vi "Actor Core.vi"(8 "error in":errorcluster, 11 "Nested in":refnum<class "FlatFieldUI.lvclass">) -> (0 "error out":errorcluster, 3 "Actor out":refnum<class "Actor.lvclass">)   [LabVIEW 2020, in "FlatField.lvlib" / "FlatFieldUI.lvlib" / "FlatFieldUI.lvclass"]
doc: "(<B>Filename</B>: Actor Framework.lvlib:Actor.lvclass:Actor Core.vi)\n\nReceives messages to the actor, reacts to them, and initiates any error handling that may shut the actor down.\n\nDescendant classes may override this VI to append parallel tasks for the actor to complete while it handles messages. Overrides use the Call Parent Method node."
uses:
  FlatFieldUI.lvclass
  C:/Program Files/National Instruments/LabVIEW 2020/vi.lib/ActorFramework/Actor/Actor.lvclass
  <vilib>/ActorFramework/Actor/Actor.lvclass
  Displayer/Displayer/FlatField Method.ctl
  FlatFieldUI.lvclass/FlatFieldUI.ctl
  <vilib>/ActorFramework/Actor/Actor.lvclass/Actor.ctl
  <vilib>/ActorFramework/Message Enqueuer/Message Enqueuer.lvclass/Message Enqueuer.ctl
  Model/Hardware Abstraction Layer/Component/Device/Device/DataExchange.ctl
  Interface/DataListener Messages/OnDataChange Msg/OnDataChange Msg.lvclass/OnDataChange Msg.ctl
  <vilib>/ActorFramework/Message Enqueuer/Init from Existing Queue.vi
  <vilib>/ActorFramework/Message Enqueuer/Enqueue.vi
  Interface/DataListener Messages/OnDataChange Msg/OnDataChange Msg.lvclass
  C:/Program Files/National Instruments/LabVIEW 2020/vi.lib/ActorFramework/Message/Message.lvclass
  <vilib>/ActorFramework/Stop Msg/Stop Msg.lvclass
  <vilib>/ActorFramework/Message Priority Queue/Priority Enqueue.vi
  <vilib>/ActorFramework/Message Enqueuer/Message Enqueuer.lvclass
  Interface/DataListener/DataListener.lvclass
  FlatField/FlatField/FlatField.lvclass
panel:
  in  "FlatFieldPath":path
  in  "DarkFieldPath":path
  in  "Save FlatField Image":bool
  in  "Save DarkField Image":bool
  in  "Method":T1 items=["Average", "Median"]
  out "Waveform Chart":dbl(graph)
  in  "Show FlatField Image":bool
  in  "Show DarkField Image":bool
  out "Frames/Dark Field":dbl
  out "Frames/Flat-Field":dbl
  in  "Frames/Flat-Field":dbl
  in  "Frames/Dark Field":dbl
  in  "TakeFlatFieldImage":bool
  in  "TakeDarkFieldImage":bool
  out "RawImage":T2(plugin-control)
  in  "Flat-Field":bool
  # "* Please Take DarkField & Flat Field Images In Live Mode\n* You need to save the DarkField/FlatField images manually for post-processing"
  # "/"
  # "1."
  # "/"
  # "2."
  # "3."
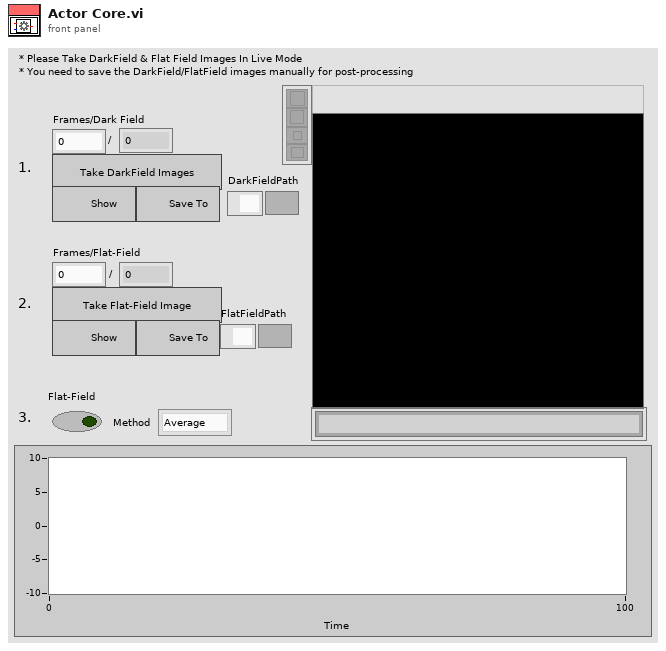
[diagram p1: front panel]
types:
  T1 = typedef "FlatField.lvlib/FlatField.lvclass/FlatField Method.ctl" = i32
  T2 = typedef "IMAQ Image.ctl" = refnum<image>
  T3 = cluster{"Stop":refnum<user-event>, "Image":refnum<user-event>}
  T4 = typedef "DataListener.lvclass/DataExchange.ctl" = cluster{"Source":string, "Destination":string, "Description":string, "value":variant}
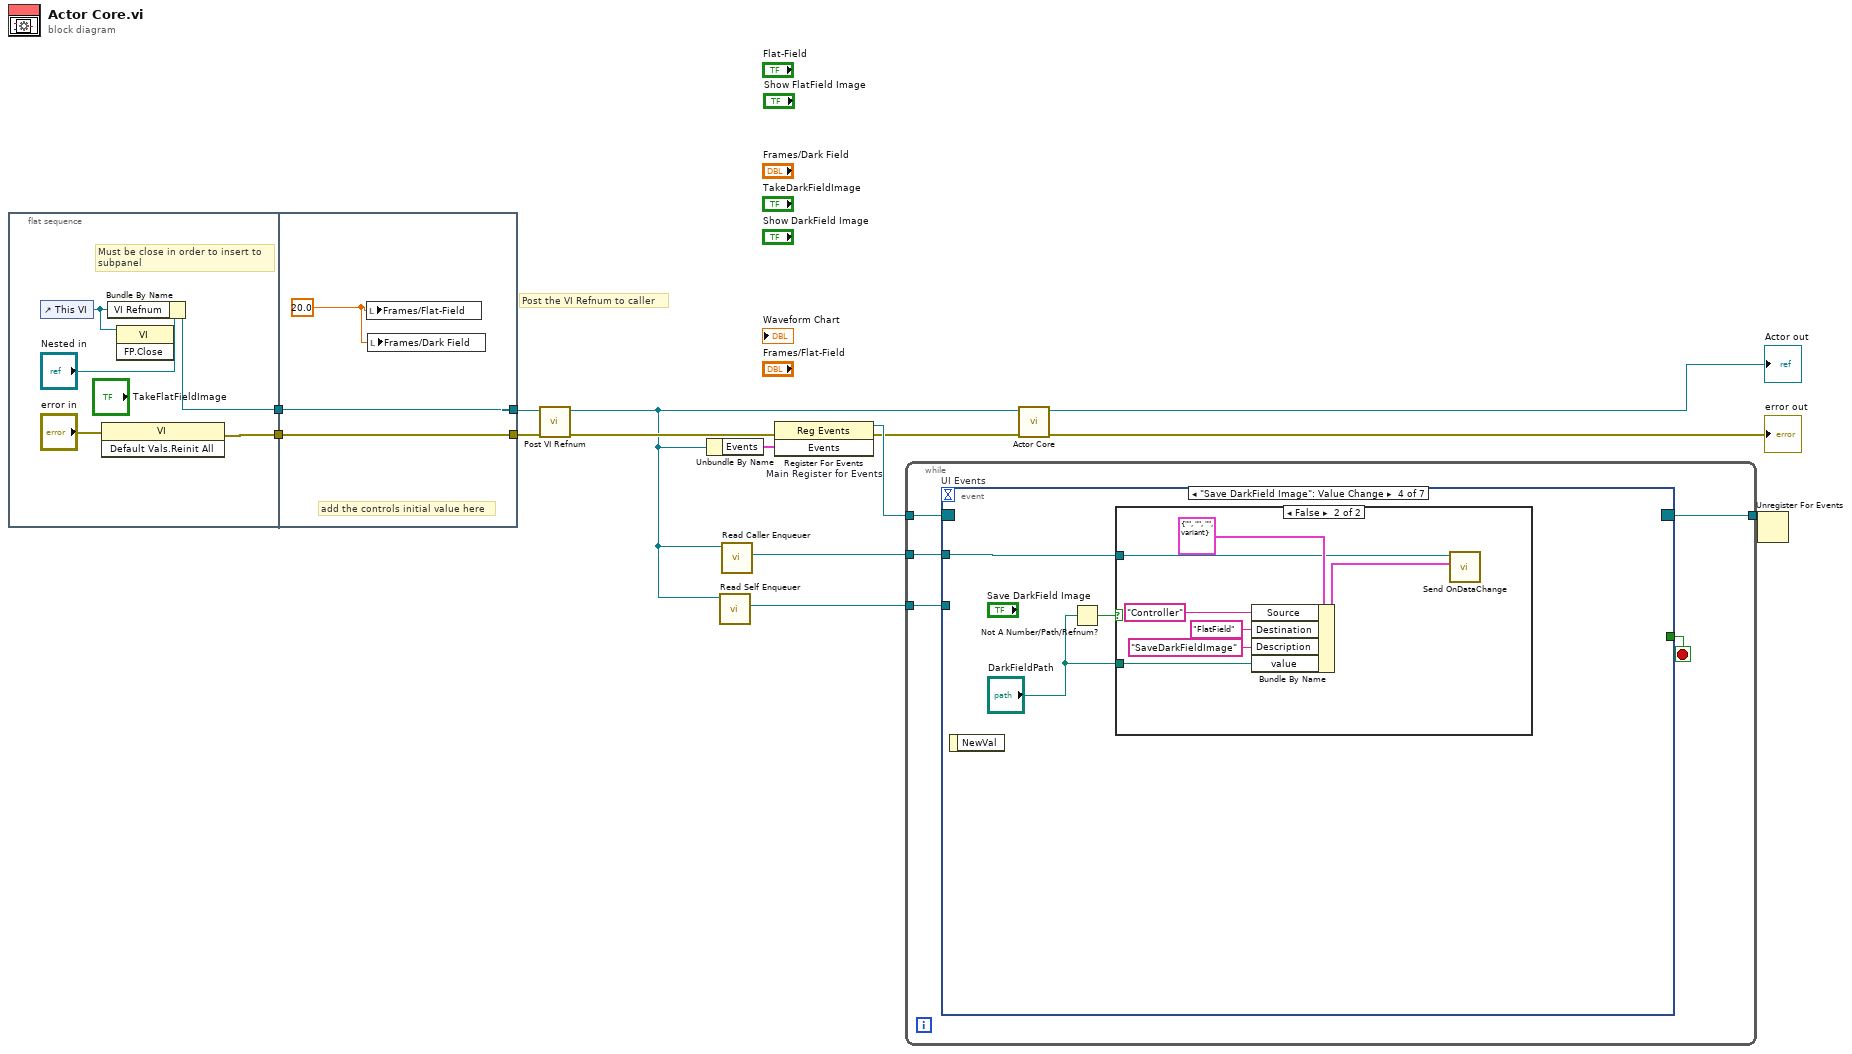
[diagram p0: block diagram]
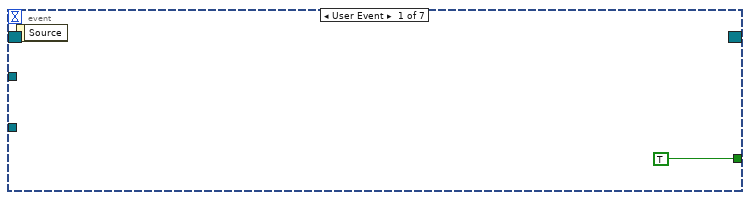
[diagram p2: hidden frame]
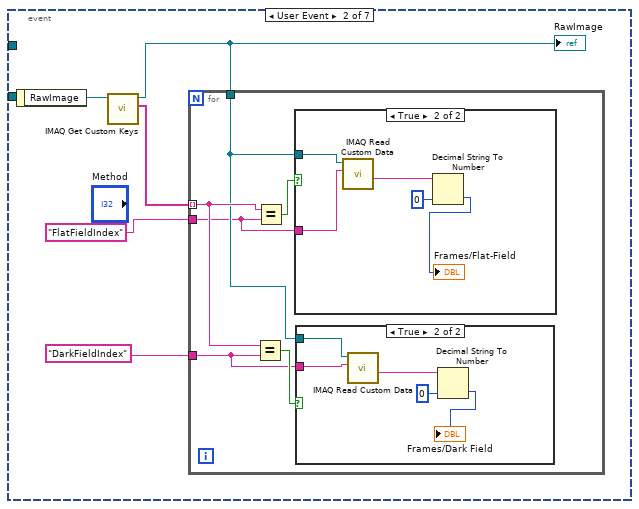
[diagram p3: hidden frame]
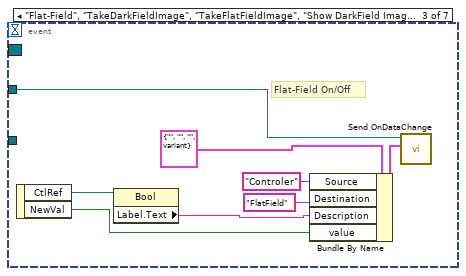
[diagram p6: hidden frame]
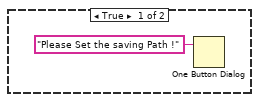
[diagram p7: hidden frame]
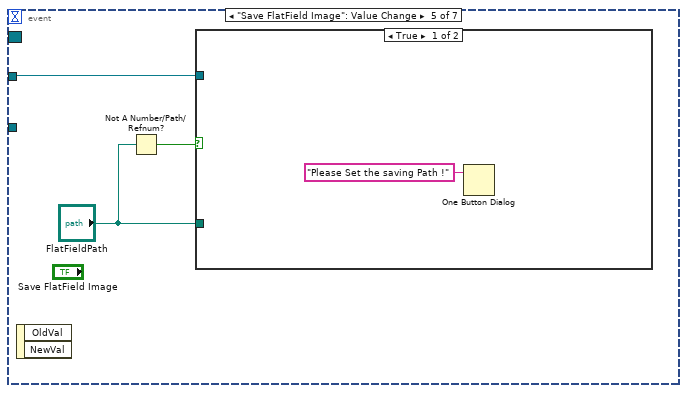
[diagram p8: hidden frame]
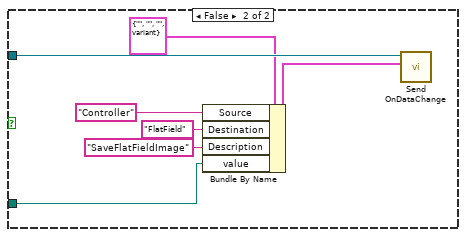
[diagram p9: hidden frame]
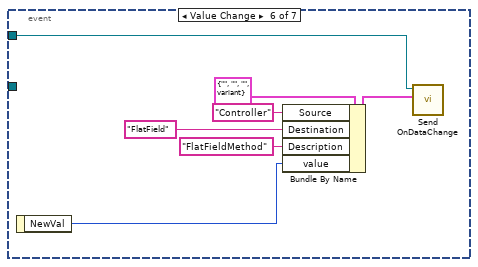
[diagram p10: hidden frame]
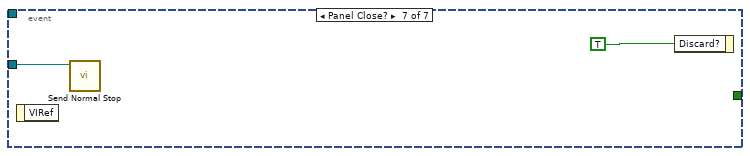
[diagram p11: hidden frame]
diagram:
  # "Post the VI Refnum to caller"
  n1 = flat-sequence {
    tunnel: [w17] -> w6
    tunnel: [w16] -> w5
    tunnel: [w21] -> w3
    tunnel: [w22] -> w7
    tunnel: w6 -> [w22]
    tunnel: w5 -> [w21]
    frame #0 {
      # "Must be close in order to insert to\nsubpanel"
      n2 = control-ref of="This VI"() -> (w15:refnum<vi>)
      n3 = invoke class="VI" method="Default Vals.Reinit All"(error in="error in") -> (error out=w17:errorcluster)  [unwired: 2 in, 2 out]
      n4 = Bundle By Name(cluster="Nested in", "VI Refnum"=w15) -> (w16:refnum<class "FlatFieldUI.lvclass">)
      n5 = invoke class="VI" method="FP.Close"(reference=w15) -> ()  [unwired: 2 in, 3 out]
    }
    frame #1 {
      w20 = 20.0 ("Frames/Flat-Field")
      # "add the controls initial value here"
      n6 = local write "Frames/Flat-Field"(w20) -> ()
      n7 = local write "Frames/Dark Field"(w20) -> ()
    }
  }
  n8 = call-dynamic "Post VI Refnum.vi"("error in (no error)"=w7, "Controller Template in"=w3) -> ("error out"=w4:errorcluster, "Controller Template out"=w2:refnum<class "FlatFieldUI.lvclass">)  [unwired: 8 in]
  n9 = Unbundle By Name(w2) -> ("Events"=w11:T3)
  n10 = call <vilib>:"Read Self Enqueuer.vi"("Actor"=w2) -> ("Self Enqueuer"=w9:refnum<class "Message Enqueuer.lvclass">)  [unwired: 10 in]
  n11 = call <vilib>:"Read Caller Enqueuer.vi"("Actor"=w2) -> ("Caller Enqueuer"=w1:refnum<class "Message Enqueuer.lvclass">)  [unwired: 10 in]
  n12 = register-events "Main Register for Events"(error in=w4, w11) -> (reference out=w12:refnum<event-registration>, error out=w8:errorcluster)  [unwired: 1 in]
  n13 = while {
    tunnel: w12 -> [w27]
    tunnel: [w25] -> w10
    tunnel: w9 -> [w24]
    tunnel: w1 -> [w23]
    stop <- w26 stop-if-true
    n14 = event "UI Events" shown="[3] \"Save DarkField Image\": Value Change" {
      selector: w27 -> [_ _ _ _ _ _ _]
      dyn-events: [_ _ _ _ _ _ _] -> w25
      timeout: _ -> [_ _ _ _ _ _ _]
      tunnel: [TRUE _ _ _ _ _ _] -> w26
      tunnel: w24 -> [_ _ _ _ _ _ w87]
      tunnel: w23 -> [_ _ w57 w60 w71 w86 _]
      event User Event {
        n15 = event-data() -> ()  [unwired: 1 in, 1 out]
      }
      event User Event {
        n16 = event-data() -> ("RawImage"=w33:T2)  [unwired: 1 in]
        n17 = call "IMAQ Get Custom Keys"("Image"=w33) -> ("Keys"=w32:string[], "Image (duplicate)"=w29:T2)  [unwired: 7 in, 2 out]
        "RawImage" <- w29
        n18 = for {
          tunnel: w32 -> [w39] mode=indexing
          tunnel: "FlatFieldIndex" ("Key") -> [w35]
          tunnel: "DarkFieldIndex" ("Key") -> [w34]
          tunnel: w29 -> [w36]
          n19 = Equal?(x=w39, y=w34) -> (x = y?=w37:bool)
          n20 = Equal?(x=w39, y=w35) -> (x = y?=w38:bool)
          n21 = case shown="True" w38 {
            tunnel: w36 -> [_ w47]
            tunnel: w35 -> [_ w46]
            frame False {
            }
            frame True {
              n22 = call "IMAQ Read Custom Data"("Key"=w46, "Image"=w47) -> ("Custom Data Out"=w49:string)  [unwired: 7 in, 2 out]
              n23 = Decimal String To Number(string=w49, default (0L)=0 ("default (0 I32)")) -> (number=→"Frames/Flat-Field":i32)  [unwired: 1 in, 1 out]
            }
          }
          n24 = case shown="True" w37 {
            tunnel: w36 -> [_ w42]
            tunnel: w34 -> [_ w41]
            frame False {
            }
            frame True {
              n25 = call "IMAQ Read Custom Data"("Key"=w41, "Image"=w42) -> ("Custom Data Out"=w43:string)  [unwired: 7 in, 2 out]
              n26 = Decimal String To Number(string=w43, default (0L)=0 ("default (0 I32)")) -> (number=→"Frames/Dark Field":i32)  [unwired: 1 in, 1 out]
            }
          }
        }
      }
      event "Flat-Field", "TakeDarkFieldImage", "TakeFlatFieldImage", "Show DarkField Image", "Show FlatField Image": Value Change {
        # "Flat-Field On/Off"
        n27 = event-data() -> ("CtlRef"=w56:refnum<vi>, "NewVal"=w50:bool)  [unwired: 1 in]
        n28 = property class="Bool"(reference=w56) -> ("Label.Text"=w51:string)  [unwired: 1 in, 2 out]
        n29 = Bundle By Name(cluster=T4 {"Source"="", "Destination"="", "Description"="", "value"=variant} ("DataExchange"), "Source"="Controler", "Destination"="FlatField", "Description"=w51, "value"=w50) -> (w54:T4)
        n30 = call "Send OnDataChange.vi"("DataExchange"=w54, "Message Enqueuer"=w57) -> ()  [unwired: 8 in, 2 out]
      }
      event "Save DarkField Image": Value Change {
        n31 = event-data() -> ()  [unwired: 1 in, 1 out]
        n32 = Not A Number/Path/Refnum?(number/path/refnum="DarkFieldPath") -> (NaN/Path/Refnum?=w59:bool)
        n33 = case shown="False" w59 {
          tunnel: w60 -> [_ w63]
          tunnel: "DarkFieldPath" -> [_ w62]
          frame True {
            n34 = One Button Dialog(message="Please Set the saving Path !") -> ()  [unwired: 1 in, 1 out]
          }
          frame False {
            n35 = Bundle By Name(cluster=T4 {"Source"="", "Destination"="", "Description"="", "value"=variant} ("DataExchange"), "Source"="Controller", "Destination"="FlatField", "Description"="SaveDarkFieldImage", "value"=w62) -> (w67:T4)
            n36 = call "Send OnDataChange.vi"("DataExchange"=w67, "Message Enqueuer"=w63) -> ()  [unwired: 8 in, 2 out]
          }
        }
      }
      event "Save FlatField Image": Value Change {
        n37 = event-data() -> ()  [unwired: 1 in, 2 out]
        n38 = Not A Number/Path/Refnum?(number/path/refnum="FlatFieldPath") -> (NaN/Path/Refnum?=w69:bool)
        n39 = case shown="True" w69 {
          tunnel: w71 -> [_ w79]
          tunnel: "FlatFieldPath" -> [_ w73]
          frame True {
            n40 = One Button Dialog(message="Please Set the saving Path !") -> ()  [unwired: 1 in, 1 out]
          }
          frame False {
            n41 = Bundle By Name(cluster=T4 {"Source"="", "Destination"="", "Description"="", "value"=variant} ("DataExchange"), "Source"="Controller", "Destination"="FlatField", "Description"="SaveFlatFieldImage", "value"=w73) -> (w77:T4)
            n42 = call "Send OnDataChange.vi"("DataExchange"=w77, "Message Enqueuer"=w79) -> ()  [unwired: 8 in, 2 out]
          }
        }
      }
      event Value Change {
        n43 = event-data() -> ("NewVal"=w83:T1)  [unwired: 1 in]
        n44 = Bundle By Name(cluster=T4 {"Source"="", "Destination"="", "Description"="", "value"=variant} ("DataExchange"), "Source"="Controller", "Destination"="FlatField", "Description"="FlatFieldMethod", "value"=w83) -> (w84:T4)
        n45 = call "Send OnDataChange.vi"("DataExchange"=w84, "Message Enqueuer"=w86) -> ()  [unwired: 8 in, 2 out]
      }
      event Panel Close? {
        n46 = event-data() -> ()  [unwired: 1 in, 1 out]
        n47 = call <vilib>:"Send Normal Stop.vi"("Message Enqueuer"=w87) -> ()  [unwired: 10 in, 1 out]
        n48 = event-data("Discard?"=TRUE) -> ()  [unwired: 1 in, 1 out]
      }
    }
  }
  n49 = call-parent "Actor Core.vi"("error in"=w8, "Actor in"=w2) -> ("error out"=→"error out":errorcluster, "Actor out"=→"Actor out":refnum<class "Actor.lvclass">)  [unwired: 8 in]
  n50 = Unregister For Events(event registration refnum=w10) -> ()  [unwired: 1 in, 1 out]
